vi "Borrar_carpeta.vi"(1 "Nº Archivos Max":i32, 2 "Path Carpeta":path) -> ()   [LabVIEW 2015]
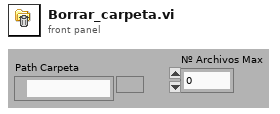
[diagram p1: front panel]
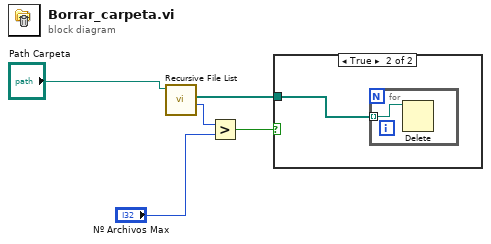
[diagram p0: block diagram]
diagram:
  n1 = call <vilib>:"Recursive File List.vi"("Folder Path"="Path Carpeta") -> ("Number of Files"=w3:i32, "All Files in Dir"=w4:path[])  [unwired: 6 in, 3 out]
  n2 = Greater?(x=w3, y="Nº Archivos Max") -> (0:w1:bool)
  n3 = case shown="True" w1 {
    tunnel: w4 -> [_ w6]
    frame False {
    }
    frame True {
      n4 = for {
        tunnel: w6 -> [w7] mode=indexing
        n5 = Delete(path (use dialog)=w7) -> ()  [unwired: 4 in, 3 out]
      }
    }
  }
